vi "Destroy Frame Buffer.vi"(8 "error in":errorcluster) -> (0 "error out":errorcluster)   [LabVIEW 2025, in "Automotive Ethernet Bus Monitor.lvclass"]
doc: "Destroy the frame buffer queue."
uses:
  Automotive Ethernet Bus Monitor.lvclass
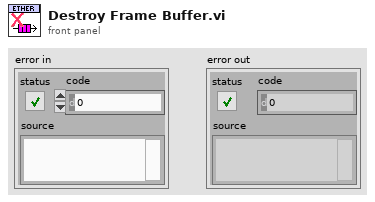
[diagram p1: front panel]
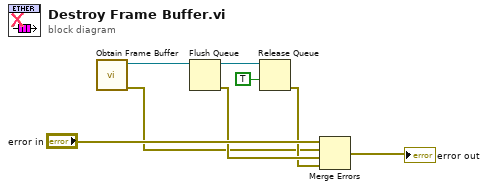
[diagram p0: block diagram]
diagram:
  n1 = call "Obtain Frame Buffer.vi"() -> ("error out"=w1:errorcluster, "queue out"=w2:refnum<queue>)  [unwired: 10 in]
  n2 = Flush Queue(queue=w2) -> (queue out=w5:refnum<queue>, error out=w4:errorcluster)  [unwired: 1 in, 1 out]
  n3 = Release Queue(queue=w5, force destroy? (F)=TRUE) -> (error out=w3:errorcluster)  [unwired: 1 in, 2 out]
  n4 = Merge Errors("error in", w1, w4, w3) -> (→"error out":errorcluster)
